vi "test_Scan Engine Sync to Scan.vi"(8 "error in (no error)":errorcluster, 11 "TestCase in":refnum<class "Scan Engine Scripting API Custom Device Unit Tests.lvclass">) -> (0 "error out":errorcluster, 3 "TestCase out":refnum<class "Scan Engine Scripting API Custom Device Unit Tests.lvclass">)   [LabVIEW 2017, in "Scan Engine Scripting API Custom Device Unit Tests.lvclass"]
uses:
  Scan Engine Scripting API Custom Device Unit Tests.lvclass
  Type Defs/Main Settings.ctl
  Scan Engine Scripting API Custom Device Unit Tests.lvclass/Scan Engine Scripting API Custom Device Unit Tests.ctl
  <vilib>/addons/_JKI Toolkits/VI Tester/TestCase.llb/TestCase.lvclass
  Scripting/Scan Engine Scripting.lvlib
  Scan Engine Custom Device.lvlib
  C:/Program Files (x86)/National Instruments/LabVIEW 2017/vi.lib/addons/_JKI Toolkits/VI Tester/TestCase.llb/TestCase.lvclass
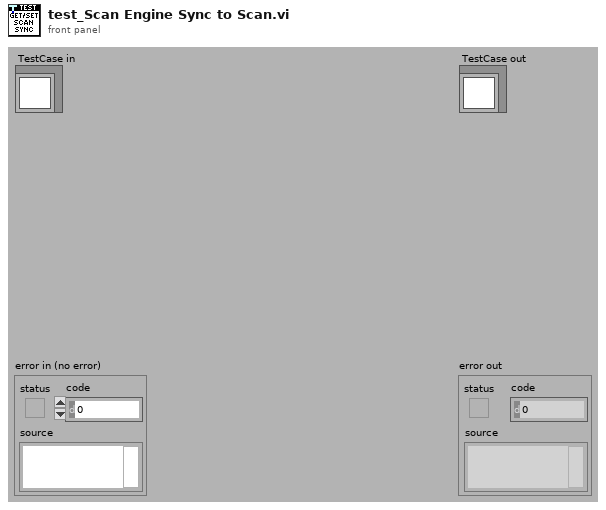
[diagram p1: front panel]
types:
  T1 = typedef "Scan Engine Custom Device.lvlib/Main Settings.ctl" = cluster{"sync to scan":bool, "scan engine decimation":u16, "delay after FPGA load (s)":u16}
  T2 = typedef "Custom Device API.lvlib/Custom Device Item Ref.ctl" = u64
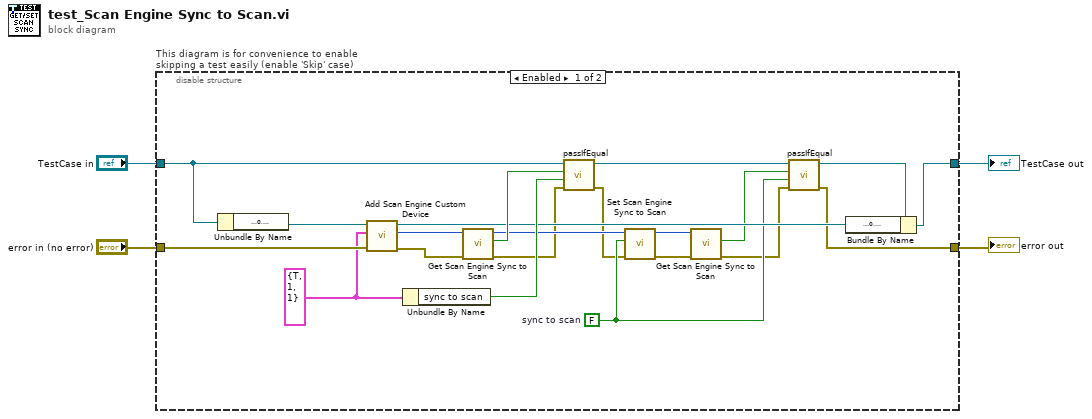
[diagram p0: block diagram]
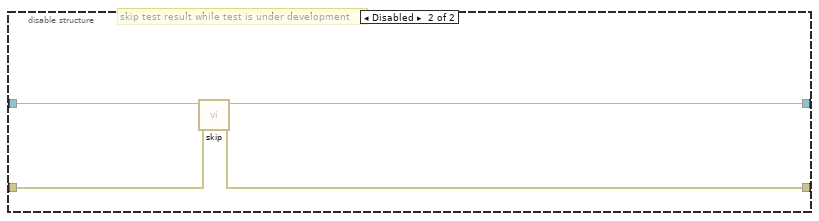
[diagram p2: hidden frame]
diagram:
  n1 = disable-structure "This diagram is for convenience to enable skipping a test easily (enable 'Skip' case)" shown="Enabled" {
    disable-tunnel: "TestCase in" -> [w23 w29]
    disable-tunnel: [w24 w27] -> w1
    disable-tunnel: [w12 w28] -> w3
    disable-tunnel: "error in (no error)" -> [w21 w26]
    frame Enabled {
      w13 = FALSE  # sync to scan
      w20 = T1 {"sync to scan"=TRUE, "scan engine decimation"=1, "delay after FPGA load (s)"=1} ("settings")
      n2 = Unbundle By Name(w23) -> ("target ref"=w22:refnum<k24>)
      n3 = call "Add Scan Engine Custom Device.vi"("error in"=w21, "settings"=w20, "target in"=w22) -> ("error out"=w10:errorcluster, "scan engine custom device ref"=w17:T2, "target out"=w16:refnum<k24>)  [unwired: 6 in]
      n4 = Unbundle By Name(w20) -> ("sync to scan"=w19:bool)
      n5 = call "Get Scan Engine Sync to Scan.vi"("error in"=w10, "scan engine custom device ref in"=w17) -> ("error out"=w9:errorcluster, "sync to scan"=w18:bool, "scan engine custom device ref out"=w15:T2)  [unwired: 7 in]
      n6 = call-dynamic "passIfEqual.vi"("error in (no error)"=w9, "y"=w19, "x"=w18, "TestCase in"=w23) -> ("error out"=w7:errorcluster, "TestCase out"=w25:refnum<class "Scan Engine Scripting API Custom Device Unit Tests.lvclass">)  [unwired: 6 in]
      n7 = call "Set Scan Engine Sync to Scan.vi"("error in"=w7, "sync to scan"=w13, "scan engine custom device ref in"=w15) -> ("error out"=w8:errorcluster, "scan engine custom device ref out"=w14:T2)  [unwired: 7 in]
      n8 = call "Get Scan Engine Sync to Scan.vi"("error in"=w8, "scan engine custom device ref in"=w14) -> ("error out"=w6:errorcluster, "sync to scan"=w5:bool)  [unwired: 7 in, 1 out]
      n9 = call-dynamic "passIfEqual.vi"("error in (no error)"=w6, "y"=w13, "x"=w5, "TestCase in"=w25) -> ("error out"=w12:errorcluster, "TestCase out"=w11:refnum<class "Scan Engine Scripting API Custom Device Unit Tests.lvclass">)  [unwired: 6 in]
      n10 = Bundle By Name(cluster=w11, "target ref"=w16) -> (w24:refnum<class "Scan Engine Scripting API Custom Device Unit Tests.lvclass">)
    }
    frame Disabled {
      # "skip test result while test is under development"
      n11 = call <vilib>:"skip.vi"("error in (no error)"=w26, "TestCase in"=w29) -> ("error out"=w28:errorcluster, "TestCase out"=w27:refnum<class "Scan Engine Scripting API Custom Device Unit Tests.lvclass">)  [unwired: 8 in]
    }
  }
  "error out" <- w3
  "TestCase out" <- w1
